vi "UpdateLimsTestStep.vi"(8 "error in (no error)":errorcluster, 10 "Step-id/Valore Prova/Tempo/Data/Udm Duration":T2, 11 "ByteGSAPIBase in":refnum<class "ByteGSAPIBase.lvclass">) -> (0 "error out":errorcluster, 2 "Result step":T1, 3 "ByteGSAPIBase out":refnum<class "ByteGSAPIBase.lvclass">)   [LabVIEW 2019, in "ByteGSWebAPI.lvlib" / "ByteGSAPIBase.lvclass"]
doc: "Update a step with the results of a simulation"
uses:
  ByteGSAPIBase.lvclass
  ByteGSAPIBase.lvclass/ByteGSAPIBase.ctl
  <vilib>/Bytelabs/ByteREST/ByteRESTClass/ByteRESTBase/RESTBase.lvclass
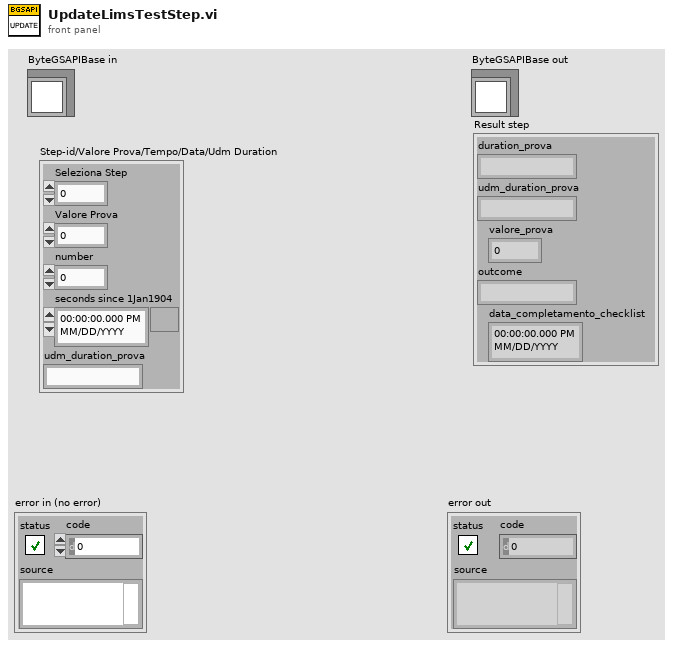
[diagram p1: front panel]
types:
  T1 = cluster{"duration_prova":string, "udm_duration_prova":string, "valore_prova":dbl, "outcome":string, "data_completamento_checklist":timestamp}
  T2 = cluster{"Seleziona Step":u16, "Valore Prova":dbl, "number":u64, "seconds since 1Jan1904":timestamp, "udm_duration_prova":string}
  T3 = cluster{"duration_prova":string, "udm_duration_prova":string, "data_completamento_checklist":string, "valore_prova":dbl, "outcome":string}
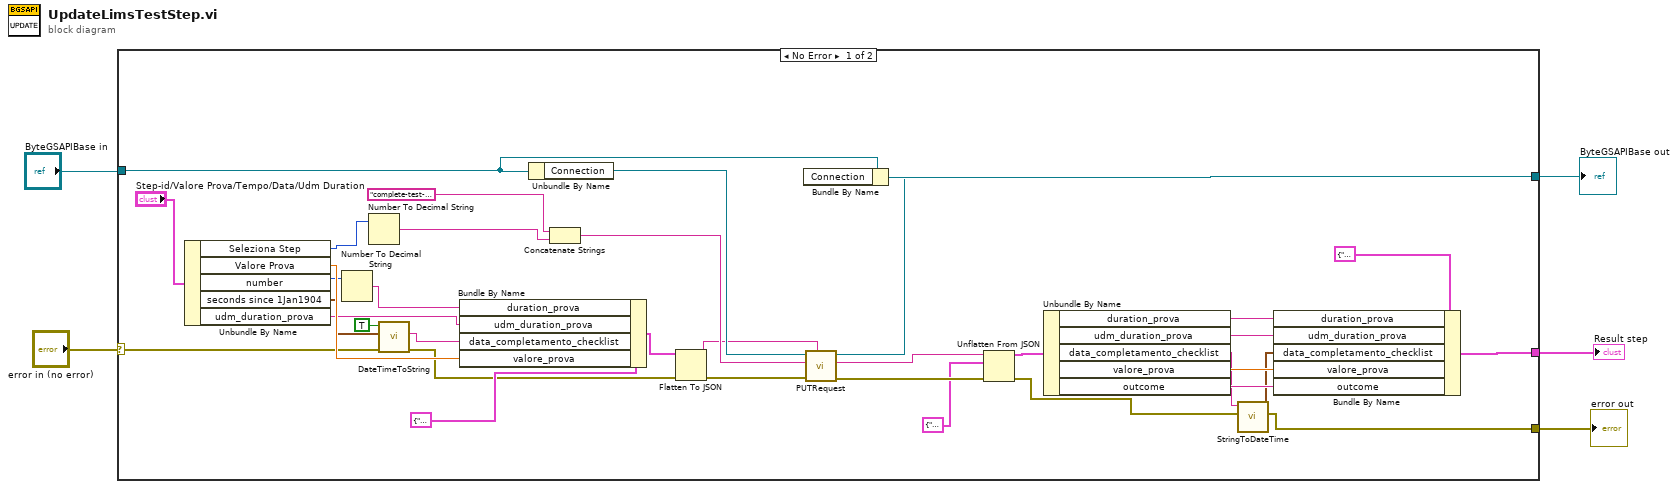
[diagram p0: block diagram]
diagram:
  n1 = case shown="No Error" "error in (no error)" {
    selector: "error in (no error)" -> [w7 w43]
    tunnel: [w10 w43] -> w4
    tunnel: [w39 w42] -> w2
    tunnel: "ByteGSAPIBase in" -> [w40 w42]
    tunnel: [w9 _] -> w1
    frame No Error {
      n2 = Unbundle By Name("Step-id/Valore Prova/Tempo/Data/Udm Duration") -> ("Seleziona Step"=w29:u16, "Valore Prova"=w26:dbl, "number"=w25:u64, "seconds since 1Jan1904"=w21:timestamp, "udm_duration_prova"=w22:string)
      n3 = Number To Decimal String(number=w25) -> (decimal integer string=w24:string)  [unwired: 1 in]
      n4 = Number To Decimal String(number=w29) -> (decimal integer string=w28:string)  [unwired: 1 in]
      n5 = call "DateTimeToString.vi"("error in"=w7, "current time"=w21, "Time"=TRUE) -> ("error out"=w8:errorcluster, "Date string"=w20:string)  [unwired: 7 in]
      n6 = Bundle By Name(cluster=T3 {"duration_prova"="3", "udm_duration_prova"="Ore", "data_completamento_checklist"="2024-10-24T17:19:12Z", "valore_prova"=5.0, "outcome"="P"} ("Update Step"), "duration_prova"=w24, "udm_duration_prova"=w22, "data_completamento_checklist"=w20, "valore_prova"=w26) -> (w23:T3)
      n7 = Unbundle By Name(w40) -> ("Connection"=w41:refnum<class "RESTBase.lvclass">)
      n8 = Concatenate Strings("complete-test-step/", w28) -> (w36:string)
      n9 = Flatten To JSON(anything=w23, error in (no error)=w8) -> (JSON string=w35:string, 11:w34:errorcluster)  [unwired: 1 in]
      n10 = call-dynamic "PUTRequest.vi"("Body in"=w35, "error in (no error)"=w34, "Request"=w36, "ByteRESTBase in"=w41) -> ("error out"=w32:errorcluster, "Body"=w33:string, "ByteRESTBase out"=w38:refnum<class "RESTBase.lvclass">)  [unwired: 4 in, 1 out]
      n11 = Bundle By Name(cluster=w40, "Connection"=w38) -> (w39:refnum<class "ByteGSAPIBase.lvclass">)
      n12 = Unflatten From JSON(JSON string=w33, type and defaults=T3 {"duration_prova"="", "udm_duration_prova"="", "data_completamento_checklist"="", "valore_prova"=0.0, "outcome"="P"}, error in (no error)=w32) -> (value=w19:T3, error out=w11:errorcluster)  [unwired: 4 in]
      n13 = Unbundle By Name(w19) -> ("duration_prova"=w17:string, "udm_duration_prova"=w16:string, "data_completamento_checklist"=w13:string, "valore_prova"=w15:dbl, "outcome"=w14:string)
      n14 = call "StringToDateTime.vi"("error in (no error)"=w11, "datetime string"=w13) -> ("error out"=w10:errorcluster, "timestamp"=w12:timestamp)  [unwired: 8 in]
      n15 = Bundle By Name(cluster=T1 {"duration_prova"="", "udm_duration_prova"="", "valore_prova"=0.0, "outcome"="P", "data_completamento_checklist"=timestamp(0 s since 1904-01-01)}, "duration_prova"=w17, "udm_duration_prova"=w16, "data_completamento_checklist"=w12, "valore_prova"=w15, "outcome"=w14) -> (w9:T1)
    }
    frame Error {
    }
  }
  "error out" <- w4
  "ByteGSAPIBase out" <- w2
  "Result step" <- w1
